vi "Set Velocity.vi"(0 "Process Variable(x)":dbl, 1 "Min Power":dbl=0.35 format="%#_13g", 2 "Max Power":dbl=0.35 format="%#_13g", 5 "Current TIme":u32, 7 "Current Power":dbl, 11 "Total Distance":dbl format="%#_13g", 12 "Last Time Input":u32) -> (4 "Coerced Motor power":dbl format="%#_13g", 6 "End Loop?":bool=TRUE, 8 "Non-Coerced Motor Power":dbl, 10 "Last Time Output":u32)   [LabVIEW 2016]
panel:
  in  "Tick range":dbl=300.0 format="%#_13g"
  in  "Power Constant (power/ms^2) constant":dbl=0.0002 format="%#_13g"
  in  "Robot Barely Moving Power":dbl=0.2 format="%#_13g"
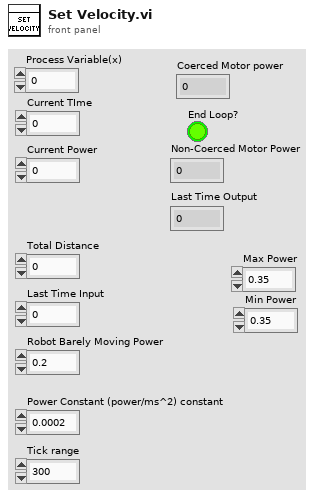
[diagram p1: front panel]
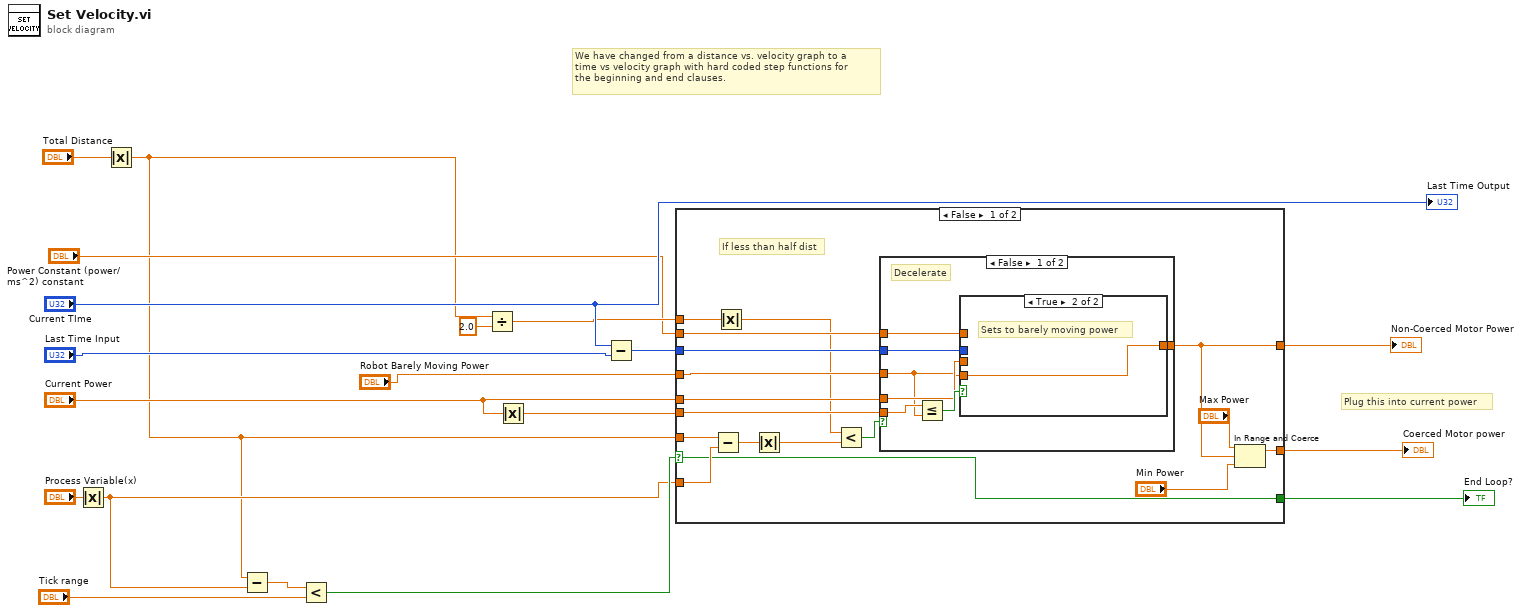
[diagram p0: block diagram]
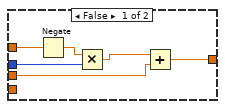
[diagram p2: hidden frame]
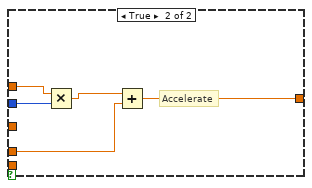
[diagram p3: hidden frame]
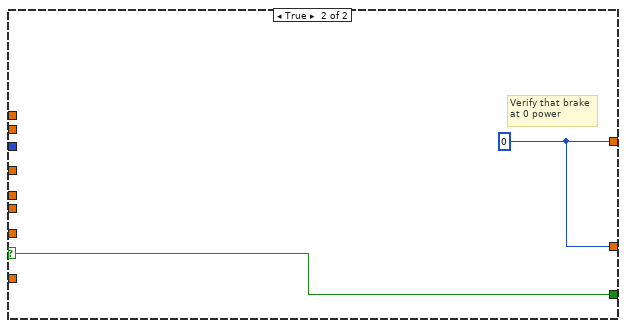
[diagram p4: hidden frame]
diagram:
  # "Plug this into current power"
  # "We have changed from a distance vs. velocity graph to a\ntime vs velocity graph with hard coded step functions for \nthe beginning and end clauses."
  n1 = Absolute Value(x="Process Variable(x)") -> (abs(x)=w2:dbl)
  n2 = Absolute Value(x="Total Distance") -> (abs(x)=w1:dbl)
  n3 = Subtract(x=w1, y=w2) -> (x-y=w3:dbl)
  n4 = Less?(x=w3, y="Tick range") -> (x < y?=w5:bool)
  n5 = Divide(x=w1, y=2.0) -> (x/y=w11:dbl)
  n6 = Absolute Value(x="Current Power") -> (abs(x)=w10:dbl)
  n7 = Subtract(x="Current TIme", y="Last Time Input") -> (x-y=w16:u32)
  n8 = case shown="False" w5 {
    selector: w5 -> [w31 w57]
    tunnel: w1 -> [w36 _]
    tunnel: w2 -> [w35 _]
    tunnel: [w33 w56] -> w19
    tunnel: [w31 w57] -> w18
    tunnel: w11 -> [w29 _]
    tunnel: "Robot Barely Moving Power" -> [w25 _]
    tunnel: w16 -> [w28 _]
    tunnel: "Current Power" -> [w23 _]
    tunnel: w10 -> [w26 _]
    tunnel: "Power Constant (power/ms^2) constant" -> [w24 _]
    tunnel: [w22 w56] -> w4
    frame False {
      # "If less than half dist"
      n9 = Subtract(x=w36, y=w35) -> (x-y=w34:dbl)
      n10 = Absolute Value(x=w29) -> (abs(x)=w21:dbl)
      n11 = Absolute Value(x=w34) -> (abs(x)=w30:dbl)
      n12 = Less?(x=w21, y=w30) -> (x < y?=w27:bool)
      n13 = case shown="False" w27 {
        tunnel: w28 -> [w39 w55]
        tunnel: [w41 w52] -> w22
        tunnel: w25 -> [w37 _]
        tunnel: w26 -> [w43 _]
        tunnel: w24 -> [w40 w54]
        tunnel: w23 -> [w38 w53]
        frame False {
          # "Decelerate"
          n14 = Less Or Equal?(x=w43, y=w37) -> (x <= y?=w42:bool)
          n15 = case shown="True" w42 {
            tunnel: [w45 w50] -> w41
            tunnel: w37 -> [_ w50]
            tunnel: w40 -> [w48 _]
            tunnel: w39 -> [w47 _]
            tunnel: w38 -> [w46 _]
            frame False {
              n16 = Negate(x=w48) -> (-x=w49:dbl)
              n17 = Multiply(x=w49, y=w47) -> (x*y=w44:dbl)
              n18 = Add(x=w44, y=w46) -> (x+y=w45:dbl)
            }
            frame True {
              # "Sets to barely moving power"
            }
          }
        }
        frame True {
          # "Accelerate"
          n19 = Multiply(x=w54, y=w55) -> (x*y=w51:dbl)
          n20 = Add(x=w51, y=w53) -> (x+y=w52:dbl)
        }
      }
      n21 = In Range and Coerce(upper limit="Max Power", x=w22, lower limit="Min Power") -> (coerced(x)=w33:dbl)  [unwired: 1 out]
    }
    frame True {
      w56 = 0
      # "Verify that brake\nat 0 power"
    }
  }
  "End Loop?" <- w18
  "Coerced Motor power" <- w19
  "Non-Coerced Motor Power" <- w4
  "Last Time Output" <- "Current TIme"
